vi "dingwei 10.23.vi"(9 "串口设置（遥控器）":T1={"波特率"=115200, "数据位"=8, "校验"=enum."None", "停止位"=10, "流控制"=0} {"流控制" items=["无"=0, "XON/XOFF"=1, "RTS/CTS"=2, "DTR/DSR"=4]; "停止位" items=["1.0"=10, "1.5"=15, "2.0"=20]; "数据位" min=5 max=8 step=1; "波特率" items=["115200"=115200, "460800"=460800, "75"=75, "110"=110, "134"=134, "150"=150, "300"=300, "600"=600, "1200"=1200, "1800"=1800, "2400"=2400, "4800"=4800, "7200"=7200, "9600"=9600, "14400"=14400, "19200"=19200, "28800"=28800, "38400"=38400, "56000"=56000, "57600"=57600, "128000"=128000, "230400"=230400]}, 11 "VISA resource name":refnum<visa-resource-name>="ASRL6::INSTR" caption="VISA资源名称") -> ()   [LabVIEW 2016]
uses:
  <vilib>/imath/engines/lvmath/Plug In/_Char/NIMS_CH_character datatype.ctl
  <vilib>/Instr/_visa.llb/VISA Configure Serial Port (Instr).vi
  <vilib>/imath/engines/lvmath2/RunTimeEngine/Managers/WorkSpace/UID Generator.vi
  <vilib>/imath/engines/lvmath/Plug In/_Char/NIMS_CH_String to Character Array.vi
  <vilib>/imath/engines/lvmath2/RunTimeEngine/BuiltInFunctions/is_empty/NIMS_is_empty(GV).vi
  <instcachedir>/0/NIMS_is_empty(GV)_FC7E7C3D9544432CB6AA2416ADCF6D56.lvgen/NIMS_is_empty(GV)_FC7E7C3D9544432CB6AA2416ADCF6D56_000.vi
  <vilib>/imath/engines/lvmath2/RunTimeEngine/BuiltInFunctions/length/NIMS_length(GV).vi
  <instcachedir>/0/NIMS_length(GV)_08A3D13377FD4E4B96F5795FBF3698FA.lvgen/NIMS_length(GV)_08A3D13377FD4E4B96F5795FBF3698FA_003.vi
  <vilib>/imath/engines/lvmath2/RunTimeEngine/RunTimeType/NIMS_RunTimeType_From StrictType (excl LVString).vi
  <instcachedir>/0/NIMS_RunTimeType_From StrictType (excl LVString)_BBF44FB49F834B71AF7A14CCEDF8BECD.lvgen/NIMS_RunTimeType_From StrictType (excl LVString)_BBF44FB49F834B71AF7A14CCEDF8BECD_000.vi
  <vilib>/imath/engines/lvmath2/RunTimeEngine/LocalVariableDefStatement/MC_LocalVariableDefStatement_Display.vi
  <vilib>/imath/engines/lvmath2/RunTimeEngine/RangeToken/NIMS_Range_R3 - Integer.vi
  <instcachedir>/0/NIMS_Range_R3 - Integer_A435E2FF893B4C718FD5055FE39FE2F6.lvgen/NIMS_Range_R3 - Integer_A435E2FF893B4C718FD5055FE39FE2F6_000.vi
  <vilib>/imath/engines/lvmath2/RunTimeEngine/CommandStatement/MC_CommandStatement_break.vi
  <vilib>/imath/engines/lvmath2/RunTimeEngine/IndexRead/NIMS M(S,S).vi
  <instcachedir>/0/NIMS M(S,S)_AC51E74150A542F7991B9634C66F3096.lvgen/NIMS M(S,S)_AC51E74150A542F7991B9634C66F3096_003.vi
  <vilib>/imathl/engines/lvmath/Functions/Error Handling/Create Error.vi
  <vilib>/imath/engines/lvmath2/RunTimeEngine/VariableToken/NIMS_VariableToken_CondDefinedDefinedByReplace.vi
  <instcachedir>/0/NIMS_VariableToken_CondDefinedDefinedByReplace_D162CFFC24174562A9FEA619A91E1A56.lvgen/NIMS_VariableToken_CondDefinedDefinedByReplace_D162CFFC24174562A9FEA619A91E1A56_003.vi
  <vilib>/imath/engines/lvmath2/RunTimeEngine/VariableToken/NIMS_VariableToken_CondDefined.vi
  <instcachedir>/0/NIMS_VariableToken_CondDefined_06E9DA95BD4D46A6BA55EC651A891960.lvgen/NIMS_VariableToken_CondDefined_06E9DA95BD4D46A6BA55EC651A891960_005.vi
  <vilib>/imath/engines/lvmath2/RunTimeEngine/IndexReplace/NIMS M(S,S)=S.vi
  <instcachedir>/0/NIMS M(S,S)=S_98E40400474E4398B113AE20298B4F82.lvgen/NIMS M(S,S)=S_98E40400474E4398B113AE20298B4F82_003.vi
  <vilib>/imath/engines/lvmath2/RunTimeEngine/ErrorHandling/NIMS_Create Error From Enums.vi
  <vilib>/imath/engines/lvmath/Plug In/_Char/NIMS_CH_Character RV to String.vi
  <vilib>/imath/engines/lvmath2/RunTimeEngine/BuiltInFunctions/findstr/NIMS_findstr.vi
  <instcachedir>/0/NIMS_length(GV)_08A3D13377FD4E4B96F5795FBF3698FA.lvgen/NIMS_length(GV)_08A3D13377FD4E4B96F5795FBF3698FA_002.vi
  <vilib>/imath/engines/lvmath2/RunTimeEngine/IndexRead/NIMS V(S).vi
  <instcachedir>/0/NIMS V(S)_0488751826AF41519A22953C041130DC.lvgen/NIMS V(S)_0488751826AF41519A22953C041130DC_002.vi
  <vilib>/imath/engines/lvmath2/RunTimeEngine/IndexRead/NIMS M(S,R2).vi
  <instcachedir>/0/NIMS M(S,R2)_45730E4D0DB74D118F715F4F99DCE4D7.lvgen/NIMS M(S,R2)_45730E4D0DB74D118F715F4F99DCE4D7_000.vi
  <instcachedir>/0/NIMS_VariableToken_CondDefined_06E9DA95BD4D46A6BA55EC651A891960.lvgen/NIMS_VariableToken_CondDefined_06E9DA95BD4D46A6BA55EC651A891960_006.vi
  <vilib>/imath/engines/lvmath2/RunTimeEngine/NodeEndStatement/NIMS_NodeEndStatement_Get Vector.vi
  <instcachedir>/0/NIMS_NodeEndStatement_Get Vector_9E4547DF38A84F62A7E036B4CE3D251C.lvgen/NIMS_NodeEndStatement_Get Vector_9E4547DF38A84F62A7E036B4CE3D251C_003.vi
  <vilib>/imath/engines/lvmath/Functions/Error Handling/MergeErrorsWrapper.vi
  <vilib>/imath/engines/lvmath2/RunTimeEngine/Managers/SymbolTable/Clear UID.vi
  <vilib>/imath/engines/lvmath2/RunTimeEngine/NodeEndStatement/NIMS_NodeEndStatement_Output.vi
  <instcachedir>/0/NIMS_NodeEndStatement_Output_53EC0D466D134D7ABD903AC30B43404B.lvgen/NIMS_NodeEndStatement_Output_53EC0D466D134D7ABD903AC30B43404B_008.vi
  <instcachedir>/0/NIMS_NodeEndStatement_Output_53EC0D466D134D7ABD903AC30B43404B.lvgen/NIMS_NodeEndStatement_Output_53EC0D466D134D7ABD903AC30B43404B_004.vi
  <instcachedir>/0/NIMS_NodeEndStatement_Output_53EC0D466D134D7ABD903AC30B43404B.lvgen/NIMS_NodeEndStatement_Output_53EC0D466D134D7ABD903AC30B43404B_011.vi
  <vilib>/imath/engines/lvmath2/RunTimeEngine/ErrorHandling/NIMS_Finalize Error.vi
  <instcachedir>/0/NIMS_is_empty(GV)_FC7E7C3D9544432CB6AA2416ADCF6D56.lvgen/NIMS_is_empty(GV)_FC7E7C3D9544432CB6AA2416ADCF6D56_001.vi
  <instcachedir>/0/NIMS M(S,S)_AC51E74150A542F7991B9634C66F3096.lvgen/NIMS M(S,S)_AC51E74150A542F7991B9634C66F3096_002.vi
  <instcachedir>/0/NIMS M(S,S)=S_98E40400474E4398B113AE20298B4F82.lvgen/NIMS M(S,S)=S_98E40400474E4398B113AE20298B4F82_002.vi
  <instcachedir>/0/NIMS_NodeEndStatement_Get Vector_9E4547DF38A84F62A7E036B4CE3D251C.lvgen/NIMS_NodeEndStatement_Get Vector_9E4547DF38A84F62A7E036B4CE3D251C_002.vi
  <vilib>/imath/engines/lvmath2/RunTimeEngine/Managers/SymbolTable/NIMS_WorkSpace.lvlib
panel:
  out "缓冲区监视器":string
  out "字节缓冲区长度":i32
  out "y":sgl format="%_6f"
  out "x":sgl format="%_6f"
  out "Zangle":sgl format="%_6f"
  in  "停止":bool
  out "PD":bool
  out "错误输出 2":errorcluster caption="错误输出"
  out "输出簇":cluster{sgl, sgl, sgl, bool}
  out "错误输出":errorcluster
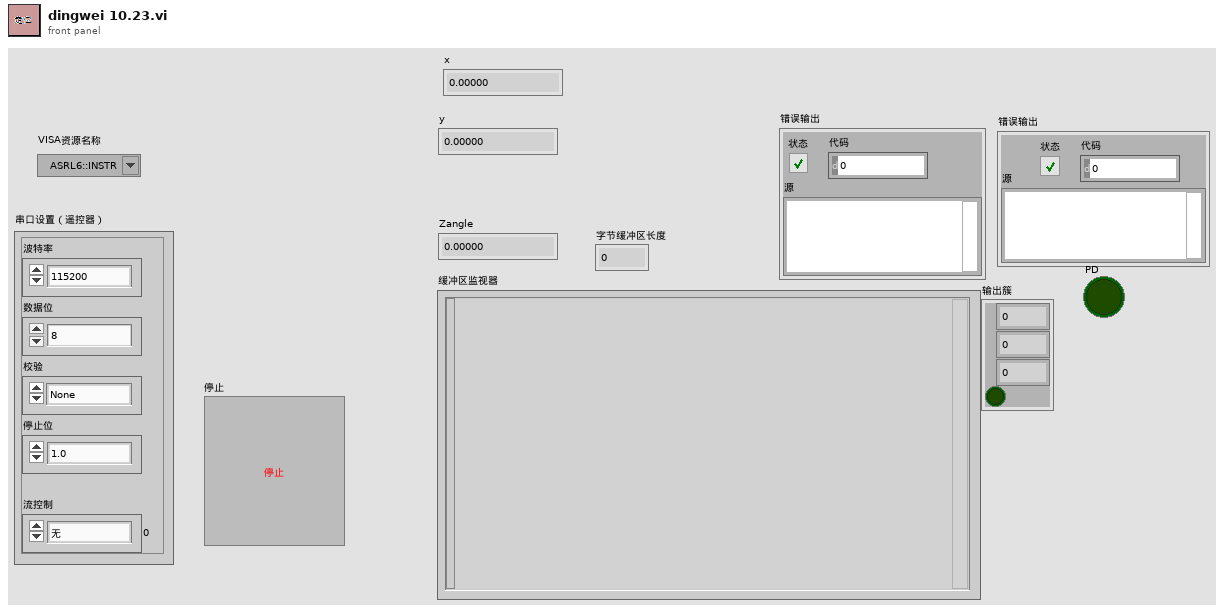
[diagram p1: front panel]
types:
  T1 = cluster{"波特率":u32, "数据位":u16, "校验":enum16{"None", "Odd", "Even", "Mark", "Space"}, "停止位":u16, "流控制":u16}
  T2 = typedef "NIMS_CH_character datatype.ctl" = cluster{"Numeric":u8}
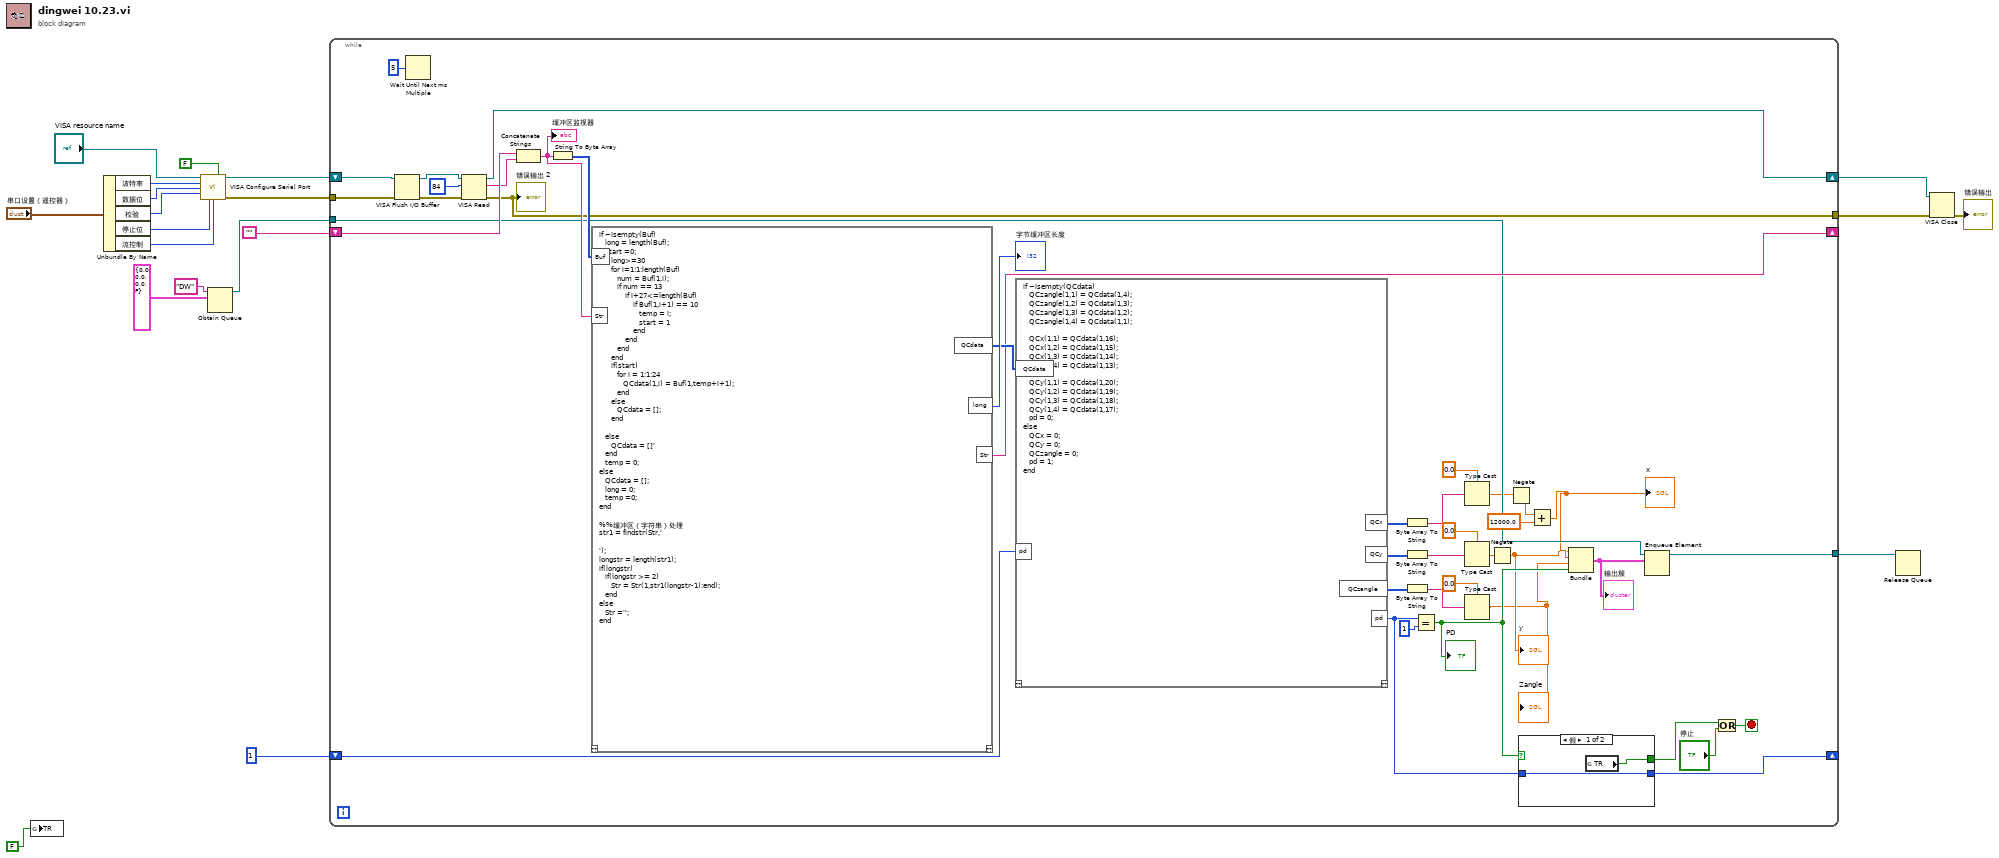
[diagram p0: block diagram]
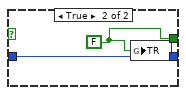
[diagram p2: hidden frame]
diagram:
  n1 = global write "全局 1.vi" "TR"(FALSE ("pr")) -> ()
  n2 = Unbundle By Name("串口设置（遥控器）") -> ("波特率"=w18:u32, "数据位"=w17:u16, "校验"=w16:enum16{"None", "Odd", "Even", "Mark", "Space"}, "停止位"=w15:u16, "流控制"=w13:u16)
  n3 = call-poly "VISA Configure Serial Port"("VISA resource name"="VISA resource name", "Enable Termination\nChar (T)"=FALSE ("Enable Termination\nChar (T)"), "baud rate (9600)"=w18, "data bits (8)"=w17, "parity (0:none)"=w16, "stop bits (10: 1 bit)"=w15, "flow control (0:none)"=w13) -> ("VISA resource name out"=w3:refnum<visa-resource-name>, "error out"=w4:errorcluster)  [unwired: 2 in, 5 out]
  n4 = Obtain Queue(name (unnamed)="DW" ("名称（未命名）"), element data type=cluster{sgl, sgl, sgl, bool} {0.0, 0.0, 0.0, FALSE} ("输出簇 2")) -> (queue out=w9:refnum<queue>)  [unwired: 3 in, 2 out]
  n5 = while {
    shift-right: [w45] -> _
    shift-left: "" -> [w62]
    shift-right: [w44] -> w11
    shift-left: w3 -> [w43]
    tunnel: [w42] -> w10
    tunnel: w9 -> [w41]
    tunnel: [w40] -> w8
    shift-right: [w30] -> _
    shift-left: 1 -> [w35]
    tunnel: w4 -> [w29]
    stop <- w38 stop-if-true
    n6 = VISA Flush I/O Buffer(VISA resource name=w43, error in (no error)=w29) -> (VISA resource name out=w46:refnum<visa-resource-name>, error out=w47:errorcluster)  [unwired: 1 in]
    n7 = Wait Until Next ms Multiple(millisecond multiple=u32 5 ("毫秒倍数")) -> ()  [unwired: 1 out]
    n8 = VISA Read(VISA resource name=w46, byte count=84, error in (no error)=w47) -> (VISA resource name out=w44:refnum<visa-resource-name>, read buffer=w61:string, error out=w42:errorcluster)  [unwired: 1 out]
    "错误输出 2" <- w42
    n9 = Concatenate Strings(w62, w61) -> (w59:string)
    "缓冲区监视器" <- w59
    n10 = String To Byte Array(string=w59) -> (unsigned byte array=w60:u8[])
    n11 = mathscript code="if ~isempty(Buf)\n   long = length(Buf);\n   start =0;\n   if long>=30\n      for i=1:1:length(Buf)\n         num = Buf(1,i);\n         if num == 13\n             if i+27<=length(Buf)\n                 if Buf(1,i+1) == 10  \n                    temp = i;\n                    start = 1\n                 end\n             end\n         end\n      end\n      if(start)\n         for i = 1:1:24\n            QCdata(1,i) = Buf(1,temp+i+1);\n         end\n      else\n         QCdata = [];\n      end\n     \n   else \n      QCdata = []'\n   end\n   temp = 0;\nelse\n   QCdata = [];\n   long = 0;\n   temp =0;\nend\n\n%%缓冲区（字符串）处理\nstr1 = findstr(Str,'\n\n');\nlongstr = length(str1);\nif(longstr)\n   if(longstr >= 2)\n      Str = Str(1,str1(longstr-1):end);\n   end\nelse\n   Str ='';\nend"("Buf"=w60, "Str"=w59) -> ("QCdata"=w57:i32[], "long"=→"字节缓冲区长度":i32, "Str"=w45:string)  [unwired: 1 in, 1 out]
    n12 = mathscript code="if ~isempty(QCdata)\n   QCzangle(1,1) = QCdata(1,4);\n   QCzangle(1,2) = QCdata(1,3);\n   QCzangle(1,3) = QCdata(1,2);\n   QCzangle(1,4) = QCdata(1,1);\n\n   QCx(1,1) = QCdata(1,16);\n   QCx(1,2) = QCdata(1,15);\n   QCx(1,3) = QCdata(1,14);\n   QCx(1,4) = QCdata(1,13);\n\n   QCy(1,1) = QCdata(1,20);\n   QCy(1,2) = QCdata(1,19);\n   QCy(1,3) = QCdata(1,18);\n   QCy(1,4) = QCdata(1,17);\n   pd = 0;\nelse \n   QCx = 0;\n   QCy = 0;\n   QCzangle = 0;\n   pd = 1;\nend"("QCdata"=w57, "pd"=w35) -> ("QCx"=w50:i32[], "QCy"=w37:i32[], "QCzangle"=w49:i32[], "pd"=w31:i32)  [unwired: 1 in, 1 out]
    n13 = Byte Array To String(unsigned byte array=w50) -> (string=w55:string)
    n14 = Byte Array To String(unsigned byte array=w37) -> (string=w53:string)
    n15 = Byte Array To String(unsigned byte array=w49) -> (string=w51:string)
    n16 = Equal?(x=w31, y=1) -> (x = y?=w33:bool)
    "PD" <- w33
    n17 = Type Cast(type=sgl 0.0, x=w55) -> (*(type *) &x=w27:sgl)
    n18 = Type Cast(type=sgl 0.0, x=w53) -> (*(type *) &x=w23:sgl)
    n19 = Type Cast(type=sgl 0.0, x=w51) -> (*(type *) &x=w21:sgl)
    "Zangle" <- w21
    n20 = Negate(x=w23) -> (-x=w22:sgl)
    "y" <- w22
    n21 = Negate(x=w27) -> (-x=w25:sgl)
    n22 = case shown="假" w33 {
      tunnel: [w63 w65] -> w34
      tunnel: w31 -> [w64 w66]
      tunnel: [w64 w66] -> w30
      frame False {
        n23 = global read "全局 1.vi" "TR"() -> (w63:bool)
      }
      frame True {
        w65 = FALSE ("pr")
        n24 = global write "全局 1.vi" "TR"(w65) -> ()
      }
    }
    n25 = Add(x=w25, y=12000.0) -> (x+y=w24:dbl)
    "x" <- w24
    n26 = Bundle(w22, w24, w21, w33) -> (w32:cluster{sgl, dbl, sgl, bool})  [unwired: 1 in]
    "输出簇" <- w32
    n27 = Enqueue Element(queue=w41, element=w32) -> (queue out=w40:refnum<queue>)  [unwired: 2 in, 2 out]
    n28 = Or(x=w34, y="停止") -> (x .or. y?=w38:bool)
  }
  n29 = Release Queue(queue=w8) -> ()  [unwired: 2 in, 3 out]
  n30 = VISA Close(VISA resource name=w11, error in (no error)=w10) -> (error out=→"错误输出":errorcluster)
